vi "Query Generation Status.vi"(8 "error in (no error)":errorcluster, 11 "AudioGeneration in":refnum<class "AudioGeneration.lvclass">) -> (0 "error out":errorcluster, 1 "timeout":bool, 2 "status":T1, 3 "AudioGeneration out":refnum<class "AudioGeneration.lvclass">)   [LabVIEW 2021, in "AudioGeneration.lvclass"]
uses:
  AudioGeneration.lvclass
  <vilib>/NI/STM/NI STM.lvlib
  <vilib>/NI/STM/TCP/Write Message (TCP).vi
  controls/generation status.ctl
  controls/AudioGenTypeDefs.lvlib
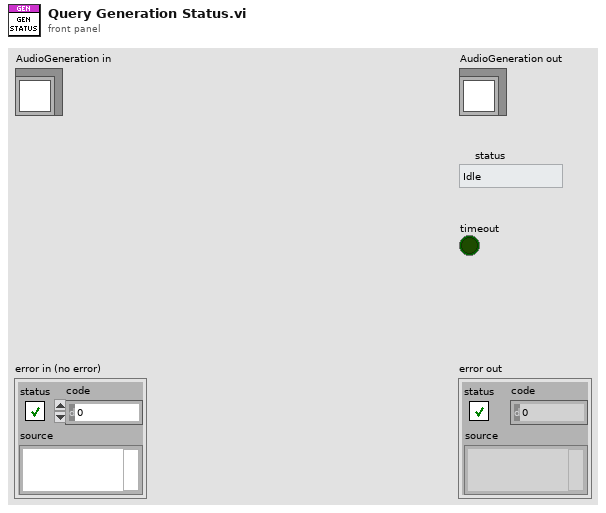
[diagram p1: front panel]
types:
  T1 = typedef "AudioGenTypeDefs.lvlib/generation status.ctl" = enum16{"Idle", "Committed", "Active"}
  T2 = typedef "AudioGenTypeDefs.lvlib/generation type.ctl" = enum16{"analog", "digital"}
  T3 = typedef "NI STM.lvlib/TCP Connection Info.ctl" = cluster{"connection ID":refnum<k5>, "meta data":T4[]}
  T4 = typedef "NI STM.lvlib/MetaDataElement.ctl" = string
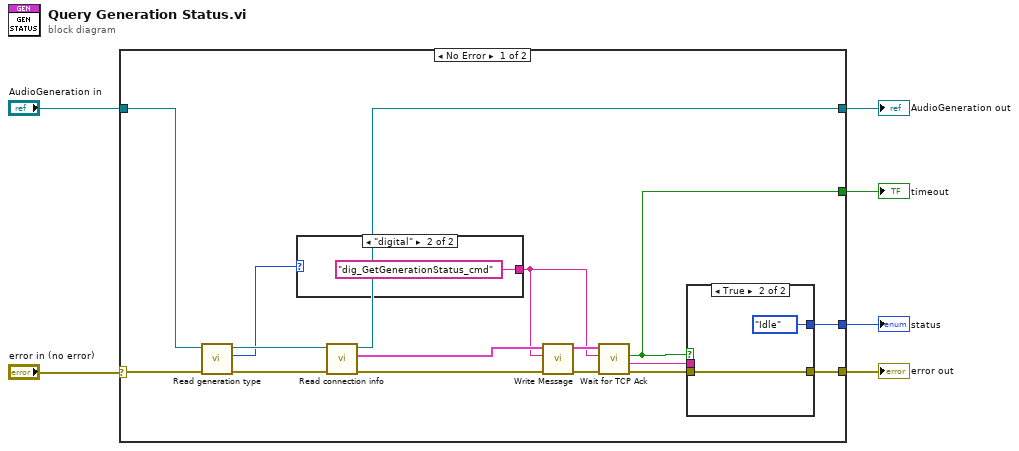
[diagram p0: block diagram]
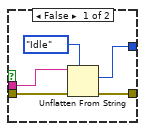
[diagram p2: hidden frame]
diagram:
  n1 = case shown="No Error" "error in (no error)" {
    selector: "error in (no error)" -> [w22 w32]
    tunnel: [w9 w32] -> w5
    tunnel: [w18 w31] -> w4
    tunnel: "AudioGeneration in" -> [w21 w31]
    tunnel: [w8 _] -> w2
    tunnel: [w7 _] -> w1
    frame No Error {
      n2 = call-dynamic "Read generation type.vi"("error in (no error)"=w22, "AudioGeneration in"=w21) -> ("error out"=w20:errorcluster, "generation type"=w17:T2, "AudioGeneration out"=w19:refnum<class "AudioGeneration.lvclass">)  [unwired: 7 in]
      n3 = case shown="\"digital\"" w17 {
        tunnel: [_ "dig_GetGenerationStatus_cmd"] -> w12
        frame "analog", Default {
        }
        frame "digital" {
        }
      }
      n4 = call-dynamic "Read connection info.vi"("error in (no error)"=w20, "AudioGeneration in"=w19) -> ("error out"=w16:errorcluster, "connection info"=w15:T3, "AudioGeneration out"=w18:refnum<class "AudioGeneration.lvclass">)  [unwired: 7 in]
      n5 = call-poly <vilib>:"Write Message.vi"("error in"=w16, "name"=w12, "connection info in"=w15) -> ("error out"=w14:errorcluster, "connection info out"=w13:T3)  [unwired: 7 in]
      n6 = call "Wait for TCP Ack.vi"("error in (no error)"=w14, "cmd name"=w12, "connection info in"=w13) -> ("error out"=w10:errorcluster, "data string"=w11:string, "timeout"=w7:bool)  [unwired: 5 in, 1 out]
      n7 = case shown="True" w7 {
        tunnel: w11 -> [w26 _]
        tunnel: w10 -> [w27 w28]
        tunnel: [w24 w28] -> w9
        tunnel: [w23 generation_status."Idle" ("status")] -> w8
        frame False {
          n8 = Unflatten From String(type=generation_status."Idle" ("status"), binary string=w26, error in (no error)=w27) -> (value=w23:T1, error out=w24:errorcluster)  [unwired: 2 in, 1 out]
        }
        frame True {
        }
      }
    }
    frame Error {
    }
  }
  "error out" <- w5
  "AudioGeneration out" <- w4
  "status" <- w2
  "timeout" <- w1
